vi "Example5.vi"() -> ()   [LabVIEW 2019]
panel:
  out "Waveform Graph":dbl[](graph)
  out "Waveform Chart":dbl(graph)
  out "Array":dbl[](array[numeric])
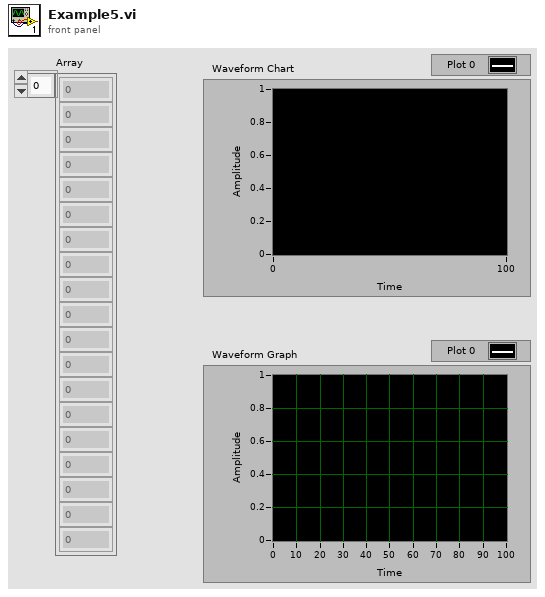
[diagram p1: front panel]
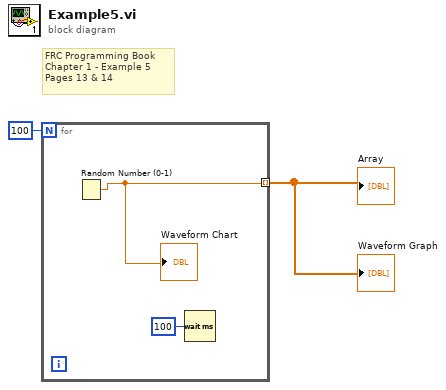
[diagram p0: block diagram]
diagram:
  # "FRC Programming Book\nChapter 1 - Example 5\nPages 13 & 14"
  n1 = for {
    N: 100 -> [_]
    tunnel: [w3] -> w1 mode=indexing
    n2 = Random Number (0-1)() -> (number: 0 to 1=w3:dbl)
    "Waveform Chart" <- w3
    n3 = Wait (ms)(milliseconds to wait=u32 100) -> ()  [unwired: 1 out]
  }
  "Array" <- w1
  "Waveform Graph" <- w1
